vi "NewCore.vi"(8 "error in (no error)":errorcluster, 10 "ParamsArray":variant[](array[variant]), 11 "NYPizzaStore":refnum<class "NYPizzaStore.lvclass">) -> (0 "error out":errorcluster, 3 "NYPizzaStore":refnum<class "NYPizzaStore.lvclass">)   [LabVIEW 2020, in "FactoryMethod.lvlib" / "PizzaFactoryMethod.lvlib" / "NYPizzaStore.lvclass"]
uses:
  NYPizzaStore.lvclass
  Private/TypeDef/privateData.ctl
  NYPizzaStore.lvclass/NYPizzaStore.ctl
  PizzaStore/PizzaStore.lvclass
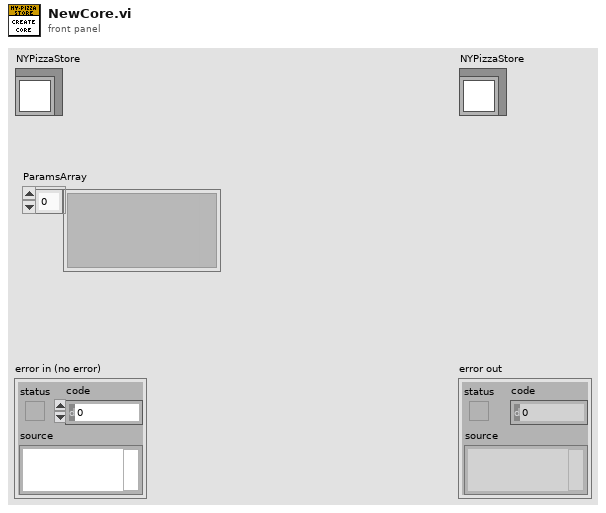
[diagram p1: front panel]
types:
  T1 = typedef "FactoryMethod.lvlib/PizzaFactoryMethod.lvlib/NYPizzaStore.lvclass/privateData.ctl" = cluster{"Dummy":i32}
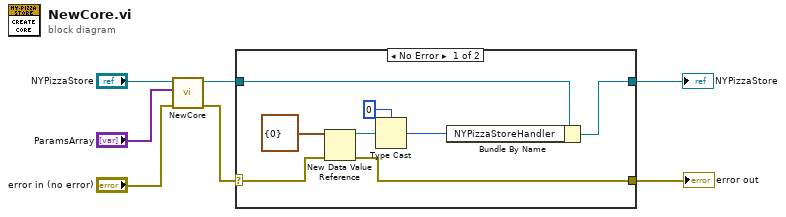
[diagram p0: block diagram]
diagram:
  n1 = call-parent "NewCore.vi"("error in (no error)"="error in (no error)", "ParamsArray"="ParamsArray", "PizzaStore"="NYPizzaStore") -> ("error out"=w2:errorcluster, "PizzaStore"=w7:refnum<class "NYPizzaStore.lvclass">)  [unwired: 7 in]
  n2 = case shown="No Error" w2 {
    selector: w2 -> [w8 w17]
    tunnel: [w10 w17] -> w5
    tunnel: [w12 w16] -> w6
    tunnel: w7 -> [w11 w16]
    frame No Error {
      n3 = New Data Value Reference(data value=T1 {"Dummy"=0} ("privateData"), error in=w8) -> (data value reference=w15:refnum<data-value>, error out=w10:errorcluster)
      n4 = Type Cast(type=u32 0, x=w15) -> (*(type *) &x=w13:u32)
      n5 = Bundle By Name(cluster=w11, "NYPizzaStoreHandler"=w13) -> (w12:refnum<class "NYPizzaStore.lvclass">)
    }
    frame Error {
    }
  }
  "error out" <- w5
  "NYPizzaStore" <- w6
